vi "QR(SubVI).vi"(8 "error in (no error)":errorcluster, 10 "New Image":T2, 11 "Refnum in":T1) -> (0 "error out":errorcluster, 1 "Data":string, 2 "Image":T2(plugin-control), 3 "Refnum out":T1, 5 "Found?":bool)   [LabVIEW 2020]
uses:
  <vilib>/userdefined/High Color/IMAQdx.ctl
  <vilib>/vision/Image Controls.llb/IMAQ Image.ctl
  <vilib>/vision/driver/NI_Vision_Acquisition_Software.lvlib
  <vilib>/vision/NI_Vision_Development_Module.lvlib
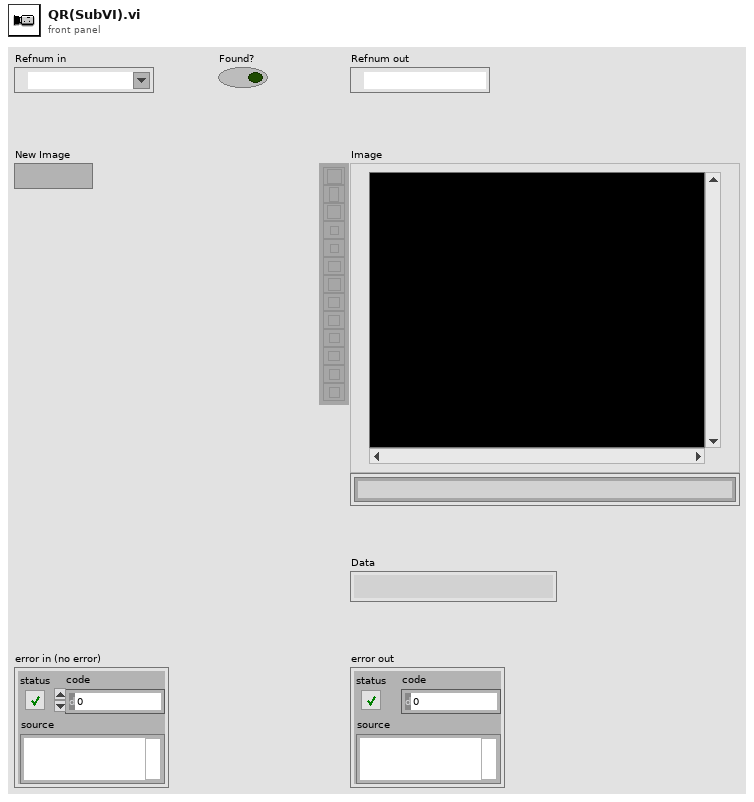
[diagram p1: front panel]
types:
  T1 = typedef "IMAQdx.ctl" = refnum<k21>
  T2 = typedef "IMAQ Image.ctl" = refnum<image>
  T3 = typedef "Image Type" = u32
  T4 = typedef "QR Code Report.ctl" = cluster{"Found?":bool, "Data":string, "Bounding Box":cluster{"x":sgl, "y":sgl}[], "Errors Corrected":u32, "Dimensions (Rows/Cols)":u32, "Version":u32, "QR Model":T5, "Stream Mode":T6, "Barcode Polarity":T7, "Mirrored?":bool, "Append Stream Position":u32, "Size of Append Stream":u32, "First EAN-128 ID":i32, "First Alternate Language ID":i32, "Append Stream ID":u32, "Minimum Edge Strength":u32, "Demodulation Mode":T8, "Cell Sample Size":T9, "Cell Filter Mode":T10}
  T5 = typedef "QR Code Model Type.ctl" = i32
  T6 = typedef "QR Code Stream Mode Type.ctl" = i32
  T7 = typedef "Data Matrix Polarity.ctl" = i32
  T8 = typedef "Demodulation Mode.ctl" = i32
  T9 = typedef "Cell Sample Size.ctl" = i32
  T10 = typedef "Cell Filter Mode.ctl" = i32
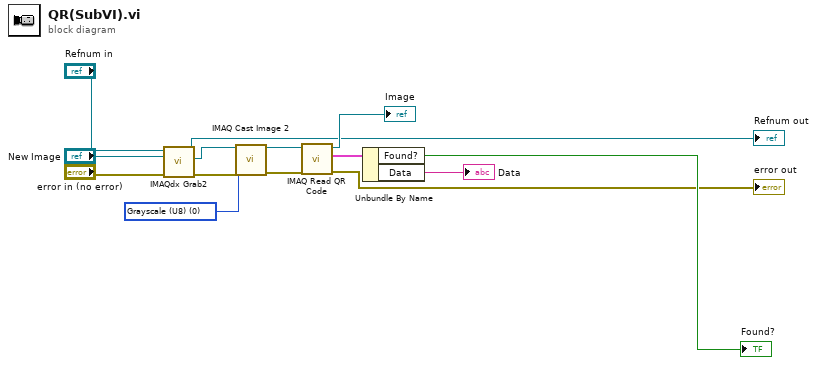
[diagram p0: block diagram]
diagram:
  w6 = T3 0 items=["Grayscale (U8)", "Grayscale (I16)", "Grayscale (SGL)", "Complex (CSG)", "RGB (U32)", "HSL (U32)", "RGB (U64)", "Grayscale (U16)"] ("Image Type")
  n1 = call <vilib>:"IMAQdx Grab2.vi"("error in"="error in (no error)", "Image In"="New Image", "Session In"="Refnum in") -> ("error out"=w5:errorcluster, "Image Out"=w4:T2, "Session Out"=→"Refnum out":T1)  [unwired: 5 in, 1 out]
  n2 = call "IMAQ Cast Image 2"("Image Src"=w4, "Image Type"=w6, "error in (no error)"=w5) -> ("Image Dst Out"=w7:T2, "error out"=w11:errorcluster)  [unwired: 11 in]
  n3 = call "IMAQ Read QR Code"("error in (no error)"=w11, "Image"=w7) -> ("error out"=→"error out":errorcluster, "QR Code Report"=w8:T4, "Image (duplicate)"=→"Image":T2)  [unwired: 6 in, 1 out]
  n4 = Unbundle By Name(w8) -> ("Found?"=→"Found?":bool, "Data"=→"Data":string)
